vi "draw sample plot.vi"(6 "Draw Area Size":cluster{"Width":u32, "Height":u32}, 7 "colors":u32[](array[colorbox])=[16717824, 16775680, 65289, 1442031, 15007983, 16746663], 8 "tout":dbl[unit][](array[numeric]), 9 "tcum":dbl[unit][](array[numeric]), 10 "State Settings":T4[][](array[typedef]) {"valve cycle time" min=0.2 step=0.1 format="%.2f"; "flow division"."5" min=0.0 max=1.0 step=0.01 format="%.3f"; "flow division"."4" min=0.0 max=1.0 step=0.01 format="%.3f"; "flow division"."3" min=0.0 max=1.0 step=0.01 format="%.3f"; "flow division"."2" min=0.0 max=1.0 step=0.01 format="%.3f"; "flow division"."1" min=0.0 max=1.0 step=0.01 format="%.3f"; "flow rate" format="%.3f"}, 11 "Samples":T7) -> (3 "Sample plot":picture)   [LabVIEW 2012]
uses:
  Samples.ctl
  State Setting.ctl
  Stamp/Switch settings vertical.ctl
  flow fraction.ctl
panel:
  in  "right white space":dbl=10.0
  in  "left white space":dbl=40.0
  out "scale specs":cluster{"coordinate":i16, "label":string}[](array[cluster])=[{"coordinate"=7, "label"="1"}, {"coordinate"=23, "label"="2"}]
  in  "scale attributes":T1={"horizontal"=TRUE, "left/top"=FALSE, "draw bar"=TRUE, "line color"=0, "text color(black)"=197379}
  in  "scale definition":T2={"coordinate 1"=0, "value 1"=0.0, "coordinate 2"=400, "value 2"=10.0, "log?(F)"=FALSE, "fmt and prec"={"format"=enum."Decimal", "precision"=0}} {"value 2" format="%0.2f"; "value 1" format="%0.2f"}
  in  "rect":T3
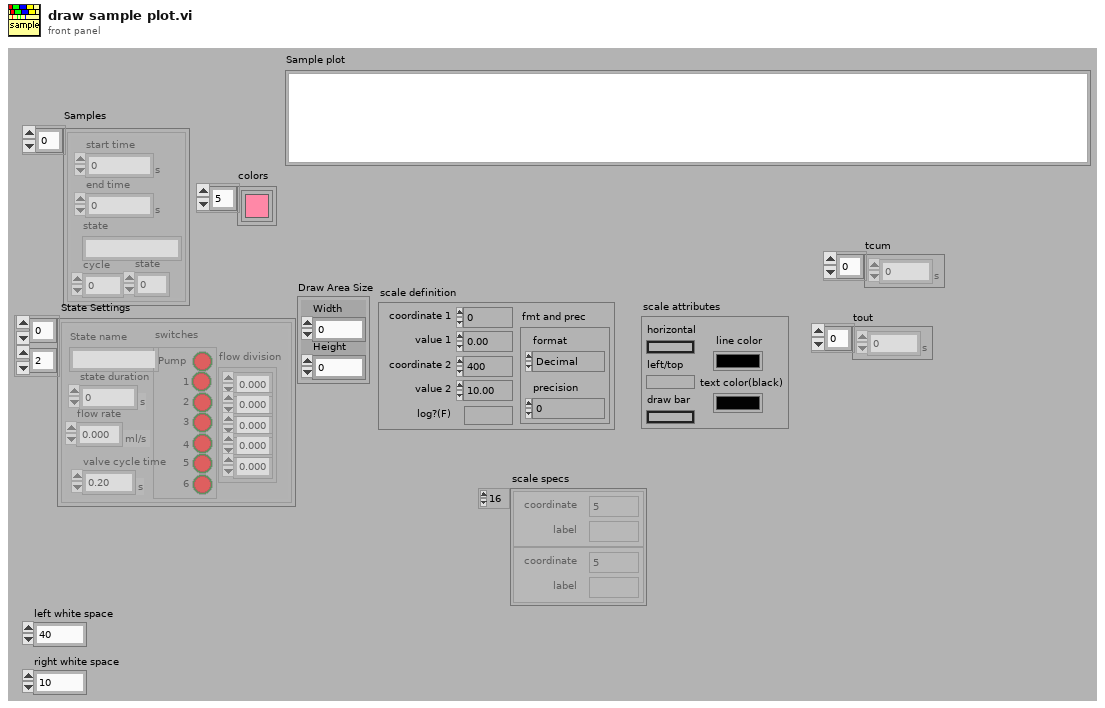
[diagram p1: front panel]
types:
  T1 = cluster{"horizontal":bool, "left/top":bool, "draw bar":bool, "line color":u32, "text color(black)":u32}
  T2 = cluster{"coordinate 1":i16, "value 1":dbl, "coordinate 2":i16, "value 2":dbl, "log?(F)":bool, "fmt and prec":cluster{"format":enum8{"Decimal", "Scientific", "Engineering", "Binary", "Octal", "Hex"}, "precision":u8}}
  T3 = cluster{"left":i16, "top":i16, "right":i16, "bottom":i16}
  T4 = typedef "State Setting.ctl" = cluster{"switches":T5, "flow rate":dbl[unit], "flow division":cluster{"1":T6, "2":T6, "3":T6, "4":T6, "5":T6}, "State name":string, "state duration":dbl[unit], "valve cycle time":dbl[unit]}
  T5 = typedef "Switch settings vertical.ctl" = cluster{"Pump":bool, "1":bool, "2":bool, "3":bool, "4":bool, "5":bool, "6":bool}
  T6 = typedef "flow fraction.ctl" = dbl
  T7 = typedef "Samples.ctl" = cluster{"start time":dbl[unit], "end time":dbl[unit], "state":string, "cycle":u16, "state":u16}[]
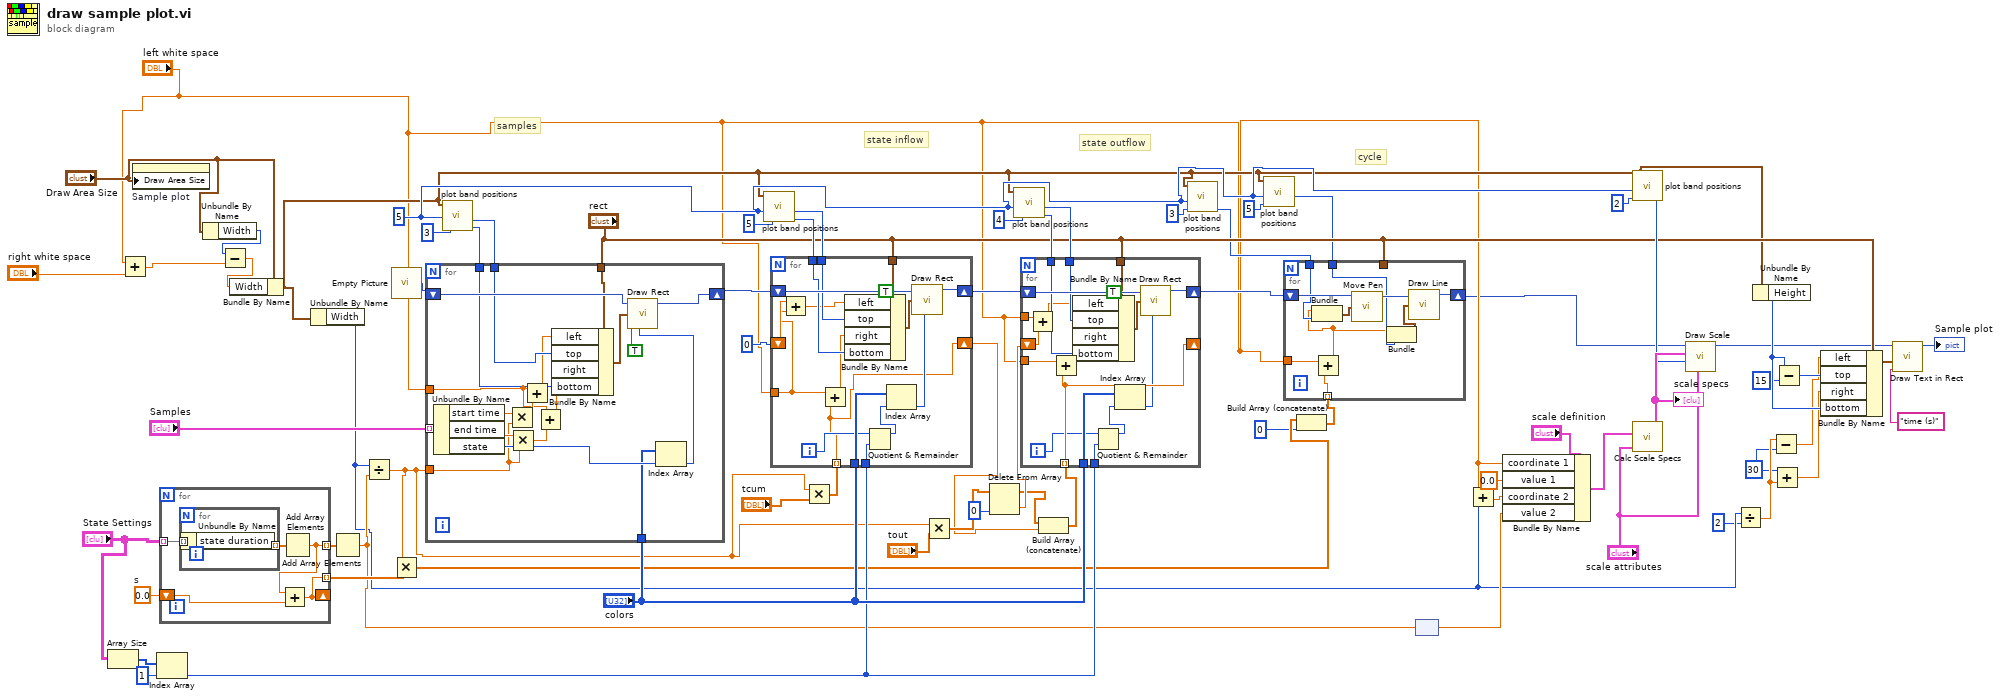
[diagram p0: block diagram]
diagram:
  w21 = u32 30 ("y")
  w33 = u32 5 ("y")
  w69 = dbl[unit] 0.0  # s
  # "cycle"
  # "state outflow"
  # "state inflow"
  # "samples"
  n1 = Array Size(array="State Settings") -> (size(s)=w65:i32[])
  n2 = Add(x="left white space", y="right white space") -> (x+y=w4:dbl)
  n3 = property on="Sample plot" class="Pict"("Draw Area Size"="Draw Area Size") -> ()  [unwired: 2 in, 2 out]
  n4 = Index Array(array=w65, index=1) -> (element=w60:i32)
  n5 = for {
    tunnel: "State Settings" -> [w78] mode=indexing
    tunnel: [w75] -> w72 mode=indexing
    tunnel: [w74] -> w70 mode=indexing
    shift-right: [w74] -> _
    shift-left: w69 -> [w76]
    n6 = for {
      tunnel: w78 -> [w80] mode=indexing
      tunnel: [w79] -> w77 mode=indexing
      n7 = Unbundle By Name(w80) -> ("state duration"=w79:dbl[unit])
    }
    n8 = Add Array Elements(numeric array=w77) -> (sum=w75:dbl[unit])
    n9 = Add(x=w75, y=w76) -> (x+y=w74:dbl[unit])
  }
  n10 = Unbundle By Name("Draw Area Size") -> ("Width"=w17:u32)
  n11 = Subtract(x=w17, y=w4) -> (x-y=w16:dbl)
  n12 = Bundle By Name(cluster="Draw Area Size", "Width"=w16) -> (w19:cluster{"Width":u32, "Height":u32})
  n13 = Unbundle By Name(w19) -> ("Width"=w28:u32)
  n14 = Add Array Elements(numeric array=w72) -> (sum=w37:dbl[unit])
  n15 = Divide(x=w28, y=w37) -> (x/y=w5:dbl[unit])
  n16 = call "Empty Picture"() -> ("empty picture"=w73:picture)
  n17 = Multiply(x=w5, y=w70) -> (x*y=w11:dbl[])
  n18 = call "plot band positions.vi"("band"=i16 3, "total bands"=w33, "Draw Area Size"=w19) -> ("bottom"=w48:u32, "top"=w49:u32)  [unwired: 2 in, 1 out]
  n19 = for {
    shift-right: [w98] -> w68
    shift-left: w73 -> [w99]
    tunnel: "Samples" -> [w97] mode=indexing
    tunnel: w5 -> [w88]
    tunnel: "rect" -> [w87]
    tunnel: "colors" -> [w86]
    tunnel: w49 -> [w85]
    tunnel: w48 -> [w84]
    tunnel: "left white space" -> [w81]
    n20 = Unbundle By Name(w97) -> ("start time"=w92:dbl[unit], "end time"=w91:dbl[unit], "state"=w95:u16)
    n21 = Multiply(x=w92, y=w88) -> (x*y=w90:dbl)
    n22 = Multiply(x=w91, y=w88) -> (x*y=w89:dbl)
    n23 = Add(x=w81, y=w90) -> (x+y=w83:dbl)
    n24 = Add(x=w81, y=w89) -> (x+y=w82:dbl)
    n25 = Bundle By Name(cluster=w87, "left"=w83, "top"=w85, "right"=w82, "bottom"=w84) -> (w96:T3)
    n26 = Index Array(array=w86, index=w95) -> (element=w94:u32)
    n27 = call <vilib>:"Draw Rect.vi"("picture"=w99, "rect"=w96, "fill?(F)"=TRUE, "color(black)"=w94) -> ("new picture"=w98:picture)  [unwired: 5 in]
  }
  n28 = call "plot band positions.vi"("band"=i16 5, "total bands"=w33, "Draw Area Size"=w19) -> ("bottom"=w45:u32, "top"=w46:u32)  [unwired: 2 in, 1 out]
  n29 = Multiply(x=w5, y="tcum") -> (x*y=w54:dbl[])
  n30 = for {
    shift-right: [w116] -> w63
    shift-left: w68 -> [w115]
    tunnel: "rect" -> [w113]
    shift-right: [w103] -> w53
    shift-left: u32 0 ("y") -> [w102]
    tunnel: w54 -> [w103] mode=indexing
    tunnel: "colors" -> [w111]
    tunnel: w60 -> [w109]
    tunnel: w46 -> [w106]
    tunnel: w45 -> [w105]
    tunnel: "left white space" -> [w100]
    i -> [w110]
    n31 = Add(x=w102, y=w100) -> (x+y=w101:dbl)
    n32 = Add(x=w100, y=w103) -> (x+y=w104:dbl)
    n33 = Bundle By Name(cluster=w113, "left"=w101, "top"=w106, "right"=w104, "bottom"=w105) -> (w114:T3)
    n34 = Quotient & Remainder(x=w110, y=w109) -> (x-y*floor(x/y)=w108:i32)  [unwired: 1 out]
    n35 = Index Array(array=w111, index=w108) -> (element=w107:u32)
    n36 = call <vilib>:"Draw Rect.vi"("picture"=w115, "rect"=w114, "fill?(F)"=TRUE, "color(black)"=w107) -> ("new picture"=w116:picture)  [unwired: 5 in]
  }
  n37 = Multiply(x=w5, y="tout") -> (x*y=w57:dbl[])
  n38 = Delete From Array(array=w57, index=0) -> (deleted portion=w56:dbl, array with subset deleted=w55:dbl[])  [unwired: 1 in]
  n39 = call "plot band positions.vi"("band"=i16 4, "total bands"=w33, "Draw Area Size"=w19) -> ("bottom"=w43:u32, "top"=w42:u32)  [unwired: 2 in, 1 out]
  n40 = Build Array (concatenate)(w55, w53) -> (w52:dbl[])
  n41 = for {
    shift-right: [w134] -> w59
    shift-left: w63 -> [w133]
    tunnel: "rect" -> [w131]
    shift-right: [w129] -> _
    shift-left: w56 -> [w130]
    tunnel: w52 -> [w129] mode=indexing
    tunnel: "colors" -> [w127]
    tunnel: w60 -> [w125]
    tunnel: w43 -> [w122]
    tunnel: w42 -> [w121]
    tunnel: "left white space" -> [w119]
    tunnel: "left white space" -> [w117]
    i -> [w126]
    n42 = Add(x=w119, y=w130) -> (x+y=w120:dbl)
    n43 = Add(x=w117, y=w129) -> (x+y=w118:dbl)
    n44 = Bundle By Name(cluster=w131, "left"=w120, "top"=w121, "right"=w118, "bottom"=w122) -> (w132:T3)
    n45 = Quotient & Remainder(x=w126, y=w125) -> (x-y*floor(x/y)=w124:i32)  [unwired: 1 out]
    n46 = Index Array(array=w127, index=w124) -> (element=w123:u32)
    n47 = call <vilib>:"Draw Rect.vi"("picture"=w133, "rect"=w132, "fill?(F)"=TRUE, "color(black)"=w123) -> ("new picture"=w134:picture)  [unwired: 5 in]
  }
  n48 = call "plot band positions.vi"("band"=i16 3, "total bands"=w33, "Draw Area Size"=w19) -> ("bottom"=w7:u32)  [unwired: 2 in, 2 out]
  n49 = call "plot band positions.vi"("band"=i16 5, "total bands"=w33, "Draw Area Size"=w19) -> ("top"=w6:u32)  [unwired: 2 in, 2 out]
  n50 = Build Array (concatenate)(w11, 0) -> (w9:dbl[])
  n51 = for {
    shift-right: [w142] -> w1
    shift-left: w59 -> [w143]
    tunnel: "rect" -> [_]
    tunnel: w9 -> [w138] mode=indexing
    tunnel: w7 -> [w140]
    tunnel: w6 -> [w137]
    tunnel: "left white space" -> [w135]
    n52 = Add(x=w135, y=w138) -> (x+y=w136:dbl)
    n53 = Bundle(w136, "bottom"=w140) -> (w141:cluster{dbl, "bottom":u32})  [unwired: 1 in]
    n54 = call <vilib>:"Move Pen.vi"("new position"=w141, "picture"=w143) -> ("new picture"=w144:picture)  [unwired: 3 in]
    n55 = Bundle(w136, "top"=w137) -> (w139:cluster{dbl, "top":u32})  [unwired: 1 in]
    n56 = call <vilib>:"Draw Line.vi"("picture"=w144, "end point"=w139) -> ("new picture"=w142:picture)  [unwired: 7 in]
  }
  n57 = node(w37) -> (w36:dbl)
  n58 = Add(x="left white space", y=w28) -> (x+y=w15:dbl)
  n59 = Bundle By Name(cluster="scale definition", "coordinate 1"="left white space", "value 1"=0.0, "coordinate 2"=w15, "value 2"=w36) -> (w39:T2)
  n60 = call "plot band positions.vi"("band"=i16 2, "total bands"=w33, "Draw Area Size"=w19) -> ("top"=w34:u32)  [unwired: 2 in, 2 out]
  n61 = call <vilib>:"Calc Scale Specs.vi"("scale definition"=w39, "scale attributes"="scale attributes") -> ("scale specs"=w51:cluster{"coordinate":i16, "label":string}[])  [unwired: 7 in]
  "scale specs" <- w51
  n62 = call <vilib>:"Draw Scale.vi"("scale attributes"="scale attributes", "constant coordinate"=w34, "scale specs"=w51, "picture"=w1) -> ("new picture"=w8:picture)  [unwired: 7 in]
  n63 = Divide(x=w28, y=u32 2) -> (x/y=w22:dbl)
  n64 = Unbundle By Name(w19) -> ("Height"=w26:u32)
  n65 = Subtract(x=w22, y=w21) -> (x-y=w20:dbl)
  n66 = Add(x=w21, y=w22) -> (x+y=w23:dbl)
  n67 = Subtract(x=w26, y=u32 15) -> (x-y=w24:u32)
  n68 = Bundle By Name(cluster="rect", "left"=w20, "top"=w24, "right"=w23, "bottom"=w26) -> (w30:T3)
  n69 = call <vilib>:"Draw Text in Rect.vi"("text"="time (s)", "rect"=w30, "picture"=w8) -> ("new picture"=→"Sample plot":picture)  [unwired: 8 in]
